vi "Group data by data type.vi"(11 "Raw data":T1) -> (1 "POI data":T1, 2 "Miniscan data":T1, 3 "Number of selected ROI per type":cluster{"# sel POI":i32, "# sel MSCN":i32})   [LabVIEW 2013]
uses:
  xcontrol/Interface VIs/Interface typedefs/Interface-Data array.ctl
  xcontrol/Interface VIs/Interface typedefs/Interface-Data format definition.ctl
  xcontrol/Typedefs/Xctl-XY data type definition.ctl
  xcontrol/Typedefs/Xctrl-ROI type enum.ctl
  Global variables/gl_Functional Imaging-Global variables.vi
  xcontrol/XGrapher.xctl
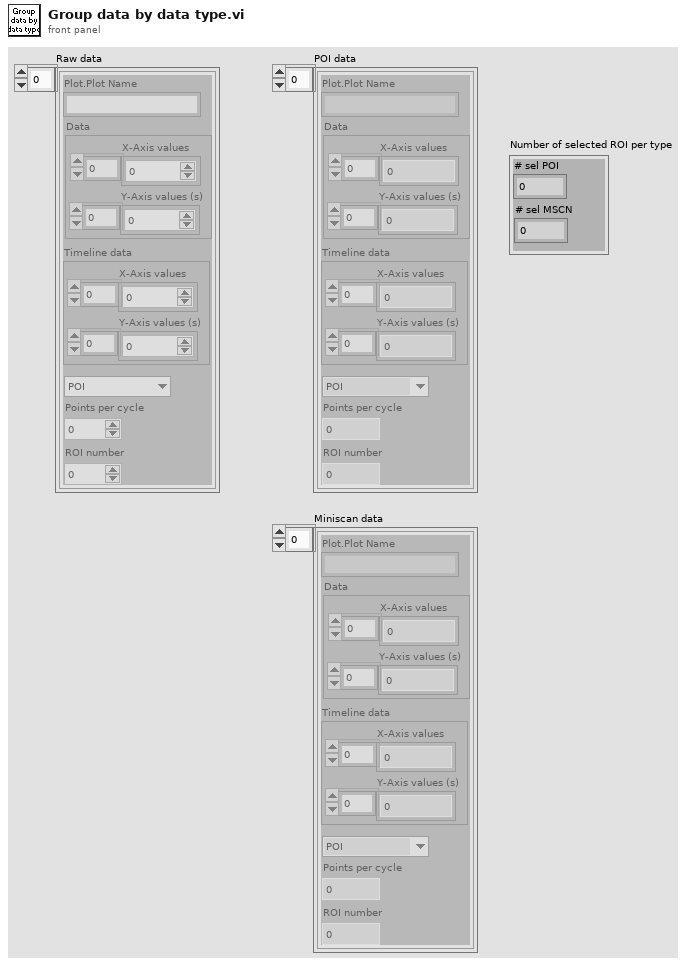
[diagram p1: front panel]
types:
  T1 = typedef "Interface-Data array.ctl" = T2[]
  T2 = typedef "Interface-Data format definition.ctl" = cluster{"Plot.Plot Name":string, "Data":T3, "Timeline data":T3, "Type":T4, "Points per cycle":u16, "ROI number":u16}
  T3 = typedef "XGrapher.xctl/Xctl-XY data type definition.ctl" = cluster{"X-Axis values":sgl[], "Y-Axis values (s)":i32[]}
  T4 = typedef "Xctrl-ROI type enum.ctl" = enum16{"POI", "Mini-scan", "Group"}
  T5 = typedef "Functional Imging UI Refs.ctl" = cluster{"Menu ref":refnum<k9>, "Image control":refnum<vi>, "VI ref":refnum<vi>, "XGrapher":refnum<vi>, "Smoothing":refnum<vi>, "POI Averaging":refnum<vi>, "Normalize":refnum<vi>, "POI data points in each trial":refnum<vi>, "Channel":refnum<vi>, "Experiment data folder path":refnum<vi>, "[ROI vis]":refnum<vi>, "[Groups] visbl":T6, "Group Name":refnum<vi>, "POI index":refnum<vi>, "Trial No.":refnum<vi>, "Intensity Zoom":refnum<vi>, "Trial Cursor Enabled":refnum<vi>, "Number of Trials (ind 1)":refnum<vi>, "Number of Trials (ind 2)":refnum<vi>, "MiniScans Available":refnum<vi>, "POI Available":refnum<vi>, "Defer graph updates":refnum<vi>, "Waveform selector":refnum<vi>, "#of selected POI":refnum<vi>, "#of selected MiniScans":refnum<vi>, "#of selected groups":refnum<vi>, "Max Z-Projection":refnum<vi>, "Z-Plane Selector":refnum<vi>, "Index of miniscan point to visualise":refnum<vi>, "ROI vis. mode":refnum<vi>, "Total # of points":refnum<vi>, "Index of group clicked on":refnum<vi>, "Pane 1":refnum<vi>, "Pane 2":refnum<vi>, "Pane 3":refnum<vi>, "Pane 4":refnum<vi>, "Pane 5":refnum<vi>, "Pane 6":refnum<vi>, "Deselect all ROI":refnum<vi>, "Deselect all groups":refnum<vi>}
  T6 = typedef "Groups array referecne.ctl" = refnum<vi>
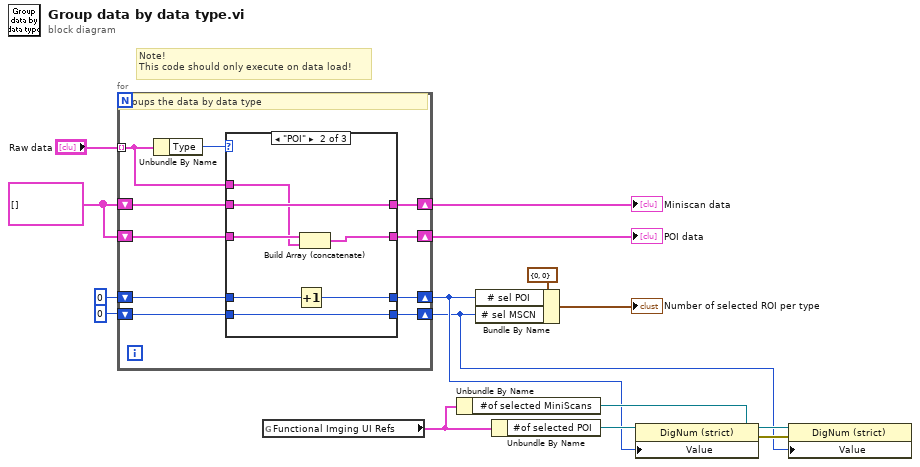
[diagram p0: block diagram]
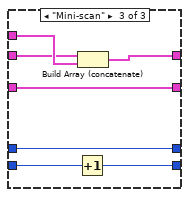
[diagram p3: hidden frame]
diagram:
  w4 = T1 [] ("Raw data out")
  # "Note!\nThis code should only execute on data load!"
  n1 = for {
    tunnel: "Raw data" -> [w22] mode=indexing
    shift-right: [w23] -> w13
    shift-left: w4 -> [w21]
    shift-right: [w20] -> w14
    shift-left: w4 -> [w19]
    shift-right: [w18] -> w6
    shift-left: 0 -> [w17]
    shift-right: [w15] -> w7
    shift-left: 0 -> [w16]
    # "Groups the data by data type"
    n2 = Unbundle By Name(w22) -> ("Type"=w24:T4)
    n3 = case shown="\"POI\"" w24 {
      tunnel: w22 -> [_ w32 w42]
      tunnel: [w27 w35 w41] -> w23
      tunnel: w21 -> [w27 w34 w41]
      tunnel: [w28 w33 w40] -> w20
      tunnel: w19 -> [w28 w33 w39]
      tunnel: [w25 w31 w38] -> w18
      tunnel: w17 -> [w25 w31 w37]
      tunnel: [w26 w29 w36] -> w15
      tunnel: w16 -> [w26 w30 w36]
      frame Default {
      }
      frame "POI" {
        n4 = Increment(x=w30) -> (x+1=w29:i32)
        n5 = Build Array (concatenate)(w34, w32) -> (w35:T1)
      }
      frame "Mini-scan" {
        n6 = Increment(x=w37) -> (x+1=w38:i32)
        n7 = Build Array (concatenate)(w39, w42) -> (w40:T1)
      }
    }
  }
  "Miniscan data" <- w14
  "POI data" <- w13
  n8 = global read "gl_Functional Imaging-Global variables.vi" "Functional Imging UI Refs"() -> (w8:T5)
  n9 = Unbundle By Name(w8) -> ("#of selected MiniScans"=w10:refnum<vi>)
  n10 = Bundle By Name(cluster=cluster{"# sel POI":i32, "# sel MSCN":i32} {"# sel POI"=0, "# sel MSCN"=0} ("Cluster"), "# sel POI"=w7, "# sel MSCN"=w6) -> (→"Number of selected ROI per type":cluster{"# sel POI":i32, "# sel MSCN":i32})
  n11 = Unbundle By Name(w8) -> ("#of selected POI"=w11:refnum<vi>)
  n12 = property on="Property Node" class="DigNum (strict)"(reference=w11, "Value"=w7) -> (error out=w9:errorcluster)  [unwired: 1 in, 1 out]
  n13 = property on="Property Node" class="DigNum (strict)"(reference=w10, error in=w9, "Value"=w6) -> ()  [unwired: 2 out]
